vi "Configure Frequency.vi"(8 "error in (no error)":errorcluster, 10 "Frequency":dbl, 11 "RS Z2X in":refnum<class "RS Z2X.lvclass">) -> (0 "error out":errorcluster, 3 "RS Z2X out":refnum<class "RS Z2X.lvclass">)   [LabVIEW 2020, in "RS Z2X.lvclass"]
doc: "Vi for configureting the frequency"
uses:
  RS Z2X.lvclass
  C:/Sandbox/Git_Sandbox/WiSpry Test Framework source code (LV20)/WiSpry Test Framework/Instruments/Instrument.lvclass
  C:/Sandbox/Git_Sandbox/WiSpry Test Framework source code (LV20)/WiSpry Test Framework/Instruments/Power Meter/Power Meter.lvclass
  Instrument.lvclass/Instrument.ctl
  Power Meter.lvclass/Power Meter.ctl
  Instrument.lvclass
  Power Meter.lvclass
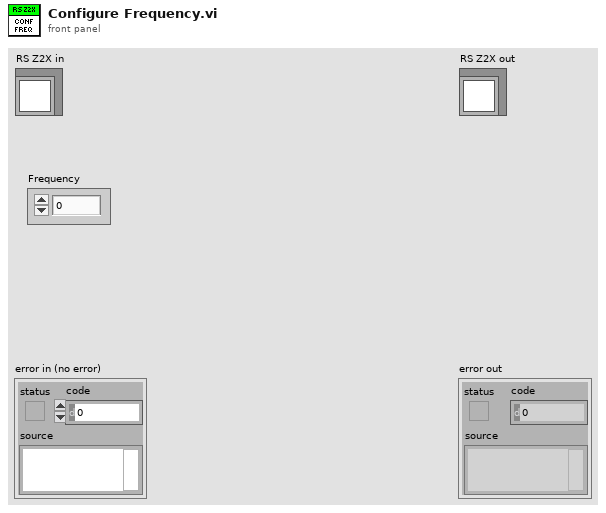
[diagram p1: front panel]
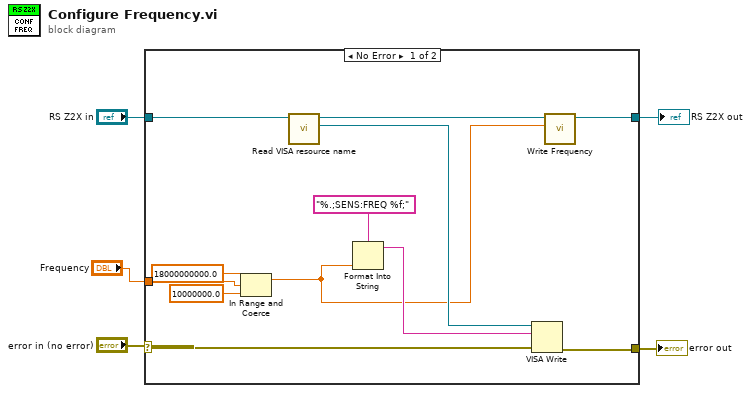
[diagram p0: block diagram]
diagram:
  n1 = case shown="No Error" "error in (no error)" {
    selector: "error in (no error)" -> [w14 w19]
    tunnel: [w16 w19] -> w2
    tunnel: "RS Z2X in" -> [w17 w18]
    tunnel: [w11 w18] -> w1
    tunnel: "Frequency" -> [w9 _]
    frame No Error {
      n2 = In Range and Coerce(upper limit=18000000000.0, x=w9, lower limit=10000000.0) -> (coerced(x)=w6:dbl)  [unwired: 1 out]
      n3 = call "Read VISA resource name.vi"("Instrument in"=w17) -> ("VISA resource name"=w15:refnum<visa-resource-name>, "Instrument out"=w10:refnum<class "RS Z2X.lvclass">)  [unwired: 9 in]
      n4 = Format Into String(format string="%.;SENS:FREQ %f;", w6) -> (resulting string=w12:string)  [unwired: 2 in, 1 out]
      n5 = VISA Write(VISA resource name=w15, write buffer=w12, error in (no error)=w14) -> (error out=w16:errorcluster)  [unwired: 2 out]
      n6 = call "Write Frequency.vi"("Frequency"=w6, "Power Meter in"=w10) -> ("Power Meter out"=w11:refnum<class "RS Z2X.lvclass">)  [unwired: 9 in]
    }
    frame Error {
    }
  }
  "error out" <- w2
  "RS Z2X out" <- w1
